vi "RT Main.vi"() -> ()   [LabVIEW 2017]
uses:
  UEFGV/Type Def/UEFGV_States.ctl
  <vilib>/event_ctls.llb/usereventprio.ctl
  programControl/programControl.lvlib
  communicateMLC/communicateMLC.lvlib
  externalAcquisition/externalAquisition.lvlib
  ErrorMonitor/ErrorMonitor.lvlib
  LowLevelController/lowLevelController.lvlib
  loggingModule/loggingModule.lvlib
panel:
  in  "stop":bool
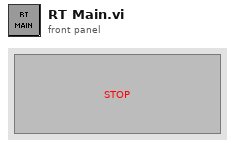
[diagram p1: front panel]
types:
  T1 = typedef "UEFGV_States.ctl" = enum16{"Create", "Get", "Destroy"}
  T2 = typedef "usereventprio.ctl" = enum32{"high priority", "normal priority"}
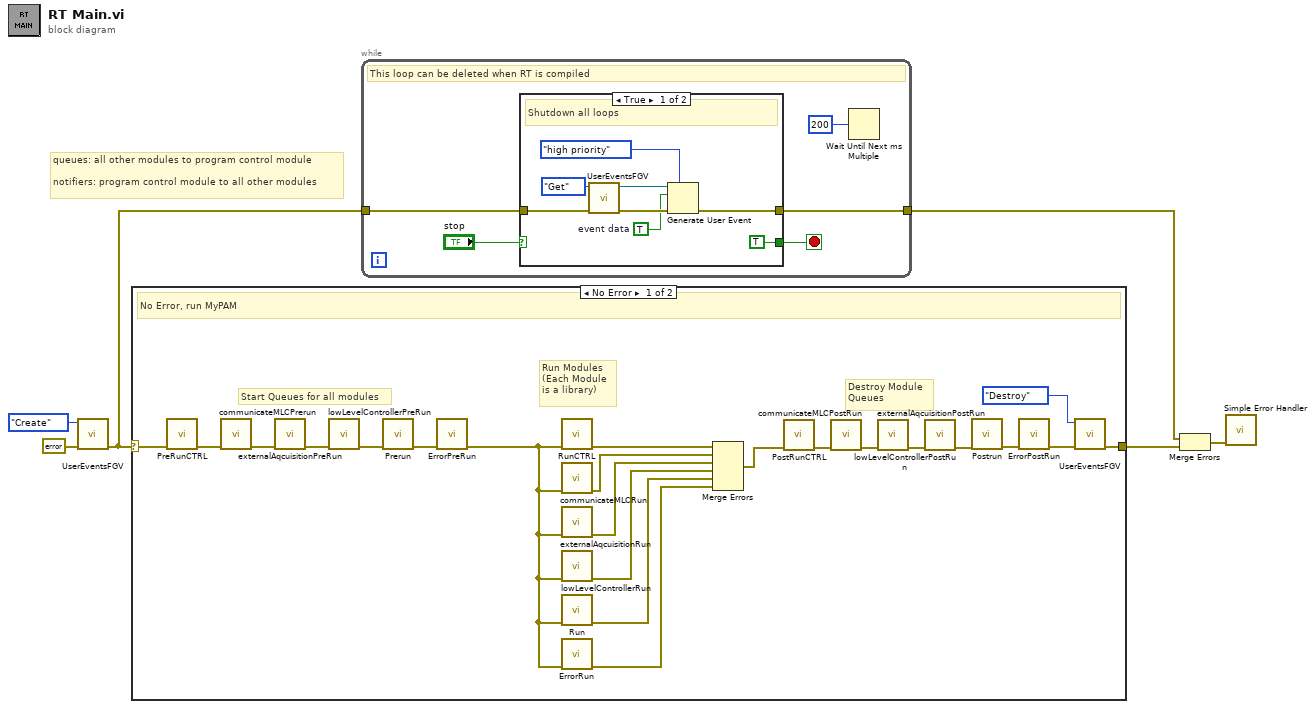
[diagram p0: block diagram]
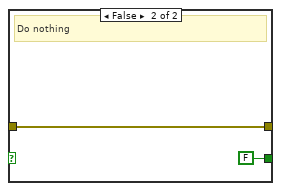
[diagram p3: hidden frame]
diagram:
  # "queues: all other modules to program control module\n\nnotifiers: program control module to all other modules"
  n1 = call "UserEventsFGV.vi"("error in (no error)"=errorcluster {"status"=FALSE, "code"=0, "source"=""} ("error constant"), "Command"=UEFGV_States."Create") -> ("error out"=w5:errorcluster)  [unwired: 8 in, 1 out]
  n2 = case shown="No Error" w5 {
    selector: w5 -> [w26 w29]
    tunnel: [w27 w29] -> w3
    frame No Error {
      # "Destroy Module\nQueues"
      # "Run Modules\n(Each Module\nis a library)"
      # "Start Queues for all modules"
      # "No Error, run MyPAM"
      n3 = call "PreRunCTRL.vi"("error in (no error)"=w26) -> ("error out"=w24:errorcluster)  [unwired: 10 in]
      n4 = call "communicateMLCPrerun.vi"("error in (no error)"=w24) -> ("error out"=w22:errorcluster)  [unwired: 10 in]
      n5 = call "externalAqcuisitionPreRun.vi"("error in (no error)"=w22) -> ("error out"=w18:errorcluster)  [unwired: 10 in]
      n6 = call "lowLevelControllerPreRun.vi"("error in (no error)"=w18) -> ("error out"=w17:errorcluster)  [unwired: 10 in]
      n7 = call "Prerun.vi"("error in (no error)"=w17) -> ("error out"=w16:errorcluster)  [unwired: 10 in]
      n8 = call "ErrorPreRun.vi"("error in (no error)"=w16) -> ("error out"=w15:errorcluster)  [unwired: 10 in]
      n9 = call "RunCTRL.vi"("error in (no error)"=w15) -> ("error out"=w25:errorcluster)  [unwired: 10 in]
      n10 = call "communicateMLCRun.vi"("error in (no error)"=w15) -> ("error out"=w23:errorcluster)  [unwired: 10 in]
      n11 = call "externalAqcuisitionRun.vi"("error in (no error)"=w15) -> ("error out"=w21:errorcluster)  [unwired: 10 in]
      n12 = call "lowLevelControllerRun.vi"("error in (no error)"=w15) -> ("error out"=w19:errorcluster)  [unwired: 10 in]
      n13 = call "Run.vi"("error in (no error)"=w15) -> ("error out"=w14:errorcluster)  [unwired: 10 in]
      n14 = call "ErrorRun.vi"("error in (no error)"=w15) -> ("error out"=w20:errorcluster)  [unwired: 10 in]
      n15 = Merge Errors(w25, w23, w21, w19, w14, w20) -> (w13:errorcluster)
      n16 = call "PostRunCTRL.vi"("error in (no error)"=w13) -> ("error out"=w12:errorcluster)  [unwired: 10 in]
      n17 = call "communicateMLCPostRun.vi"("error in (no error)"=w12) -> ("error out"=w11:errorcluster)  [unwired: 10 in]
      n18 = call "externalAqcuisitionPostRun.vi"("error in (no error)"=w11) -> ("error out"=w10:errorcluster)  [unwired: 10 in]
      n19 = call "lowLevelControllerPostRun.vi"("error in (no error)"=w10) -> ("error out"=w9:errorcluster)  [unwired: 10 in]
      n20 = call "Postrun.vi"("error in (no error)"=w9) -> ("error out"=w8:errorcluster)  [unwired: 10 in]
      n21 = call "ErrorPostRun.vi"("error in (no error)"=w8) -> ("error out"=w7:errorcluster)  [unwired: 10 in]
      n22 = call "UserEventsFGV.vi"("error in (no error)"=w7, "Command"=UEFGV_States."Destroy") -> ("error out"=w27:errorcluster)  [unwired: 8 in, 1 out]
    }
    frame Error {
      # "Error, DO NOT RUN"
    }
  }
  n23 = while {
    tunnel: w5 -> [w31]
    tunnel: [w30] -> w2
    stop <- w32 stop-if-true
    # "This loop can be deleted when RT is compiled"
    n24 = case shown="True" "stop" {
      tunnel: [TRUE FALSE] -> w32
      tunnel: w31 -> [w41 w43]
      tunnel: [w38 w43] -> w30
      frame True {
        w36 = TRUE  # event data
        # "Shutdown all loops"
        n25 = call "UserEventsFGV.vi"("error in (no error)"=w41, "Command"=UEFGV_States."Get") -> ("error out"=w40:errorcluster, "Shutdown User Event"=w39:refnum<user-event>)  [unwired: 8 in]
        n26 = Generate User Event(priority (normal)=usereventprio."high priority", user event=w39, event data cluster=w36, error in=w40) -> (error out=w38:errorcluster)  [unwired: 1 out]
      }
      frame False {
        # "Do nothing"
      }
    }
    n27 = Wait Until Next ms Multiple(millisecond multiple=u32 200) -> ()  [unwired: 1 out]
  }
  n28 = Merge Errors(w2, w3) -> (w1:errorcluster)
  n29 = call <vilib>:"Simple Error Handler.vi"("error in (no error)"=w1) -> ()  [unwired: 4 in, 5 out]
